vi "Wavelength.vi"(8 "error in (no error)":errorcluster, 10 "Spectrometer Triax 550.lvclass":refnum<class "Spectrometer Triax 550.lvclass">, 11 "Wavelength in":refnum<class "Wavelength.lvclass">) -> (0 "error out":errorcluster, 3 "Wavelength out":refnum<class "Wavelength.lvclass">)   [LabVIEW 2015, in "Wavelength.lvclass"]
uses:
  Wavelength.lvclass
  Instruments/Spectrometer/Spectrometer Triax 550.lvclass
  Scanner/Scanner.lvclass
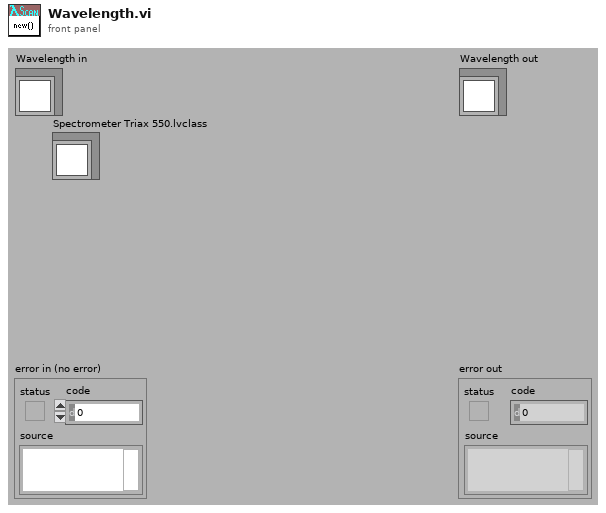
[diagram p1: front panel]
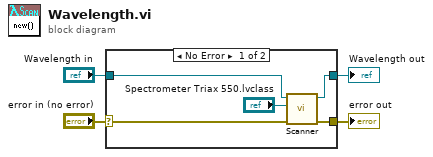
[diagram p0: block diagram]
diagram:
  n1 = case shown="No Error" "error in (no error)" {
    selector: "error in (no error)" -> [w7 w11]
    tunnel: [w6 w11] -> w3
    tunnel: [w8 w10] -> w1
    tunnel: "Wavelength in" -> [w9 w10]
    frame No Error {
      n2 = call "Scanner.vi"("error in (no error)"=w7, "Scannable"="Spectrometer Triax 550.lvclass", "Scanner.lvclass in"=w9) -> ("error out"=w6:errorcluster, "Scanner.lvclass out"=w8:refnum<class "Wavelength.lvclass">)  [unwired: 1 in, 6 out]
    }
    frame Error {
    }
  }
  "error out" <- w3
  "Wavelength out" <- w1
